vi "DCA Calibration Dialog.vi"(6 "Driver Refs":T4, 8 "error in (no error)":errorcluster, 11 "Current Calibration":T1) -> (0 "error out":errorcluster, 3 "Calibration Out":T1, 4 "Driver Refs Out":T4)   [LabVIEW 2011]
uses:
  drivers/DMM/DMM Driver Ref.ctl
  drivers/SWI/SWI Driver Ref.ctl
  TypeDefs/DCA Calibration State.ctl
  drivers/DMM/DMM Measurement.ctl
  drivers/DMM/DMM Command.ctl
  drivers/SWI/SWI Command.ctl
panel:
  out "Rbc Indicator":cluster{"Pass":bool, "Fail":bool}
  out "Rac Indicator":cluster{"Pass":bool, "Fail":bool}
  out "Rab Indicator":cluster{"Pass":bool, "Fail":bool}
  in  "Clear":bool
  in  "Rbc":bool
  in  "Rac":bool
  in  "Rab":bool
  in  "Done":bool
  in  "Message (\"\")":string="The instrument is ready for normalization.\n\nPlease insert the appropriate shorts into the test fixture and select one of the following options:\n\n    Rab  -  calibrate the Rab switch position.\n    Rac  -  calibrate the Rac switch position.\n    Rbc  -  calibrate the Rbc switch position.\n    Done  -  accept the normalization offsets and continue testing by\n                  following these steps:\n                     1)  Remove the short from the test fixtrue;\n                     2)  Place the part to be measured into the test fixture;\n                     3)  Press the Done button to continue."
  out "Cal Header":string="Normalization Offsets:\n\nRab = 0.00\nRac = 0.00\nRbc = 0.00"
  out "Cal Accepted?":bool
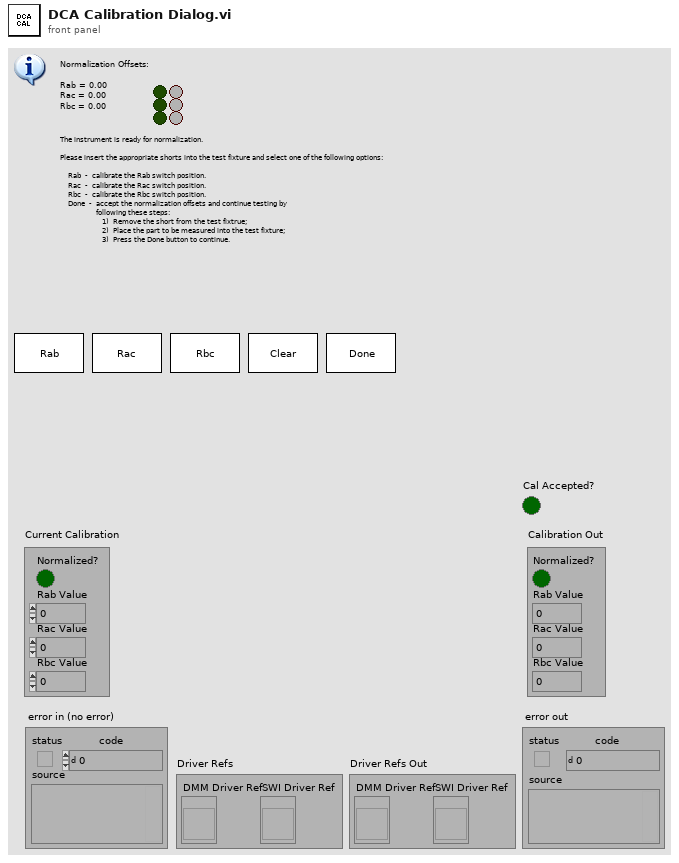
[diagram p1: front panel]
types:
  T1 = typedef "DCA Calibration State.ctl" = cluster{"Normalized?":bool, "Rab Value":dbl, "Rac Value":dbl, "Rbc Value":dbl}
  T2 = typedef "DMM Driver Ref.ctl" = refnum<vi>
  T3 = typedef "SWI Driver Ref.ctl" = refnum<vi>
  T4 = cluster{"DMM Driver Ref":T2, "SWI Driver Ref":T3}
  T5 = typedef "DMM Measurement.ctl" = dbl
  T6 = typedef "DMM Command.ctl" = enum16{"LOAD", "INITIALIZE", "PRESET", "GET STIMULUS", "SET STIMULUS", "MEASURE", "RELEASE", "UNLOAD", "GET CALIBRATION", "CALIBRATE"}
  T7 = typedef "SWI Command.ctl" = enum16{"LOAD", "INITIALIZE", "PRESET", "SET STIMULUS", "GET STIMULUS", "GET INFO", "RELEASE", "UNLOAD"}
  T8 = typedef "Sea-Level SWI Position.ctl" = cluster{"Port 1 (0)":cluster{"0":bool, "1":bool, "2":bool, "3":bool, "4":bool, "5":bool, "6":bool, "7":bool}, "Port 2 (1)":cluster{"0":bool, "1":bool, "2":bool, "3":bool, "4":bool, "5":bool, "6":bool, "7":bool}, "Port 3 (2)":cluster{"0":bool, "1":bool, "2":bool, "3":bool, "4":bool, "5":bool, "6":bool, "7":bool}, "Port 4 (3)":cluster{"0":bool, "1":bool, "2":bool, "3":bool, "4":bool, "5":bool, "6":bool, "7":bool}}
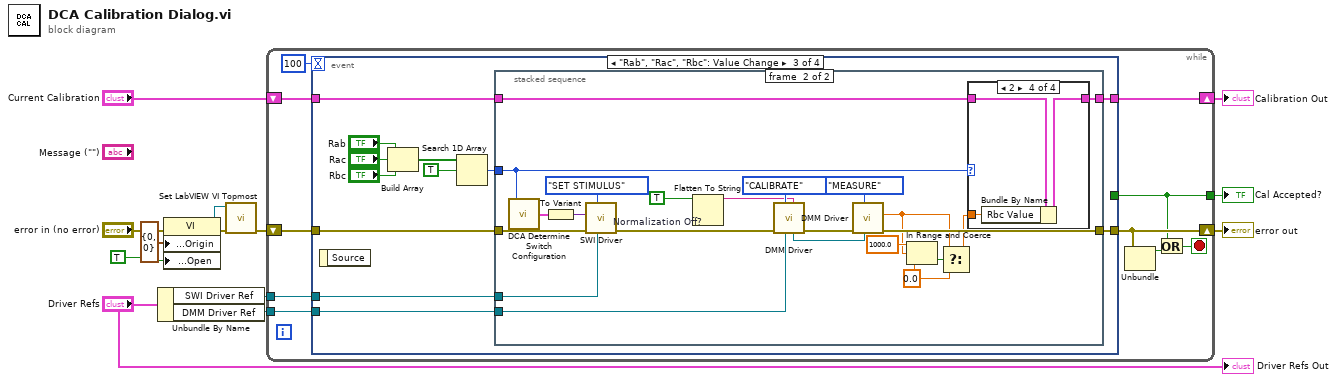
[diagram p0: block diagram]
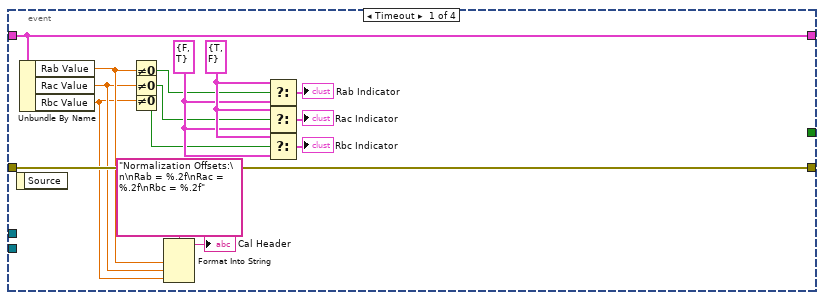
[diagram p2: hidden frame]
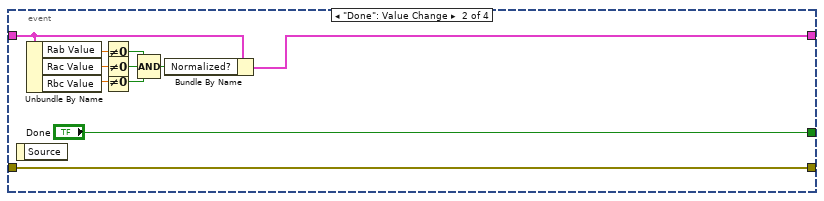
[diagram p3: hidden frame]
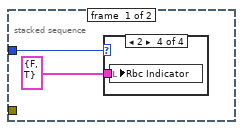
[diagram p4: hidden frame]
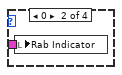
[diagram p6: hidden frame]
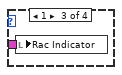
[diagram p7: hidden frame]
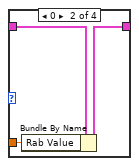
[diagram p9: hidden frame]
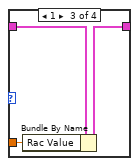
[diagram p10: hidden frame]
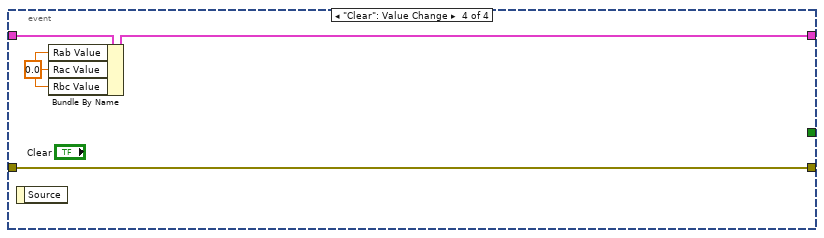
[diagram p11: hidden frame]
diagram:
  n1 = Unbundle By Name("Driver Refs") -> ("SWI Driver Ref"=w11:T3, "DMM Driver Ref"=w10:T2)
  n2 = property on="Property Node" class="VI"(error in="error in (no error)", "Front Panel Window:Origin"=cluster{"Horizontal":i16, "Vertical":i16} {"Horizontal"=0, "Vertical"=0}, "Front Panel Window:Open"=TRUE) -> (reference out=w6:refnum<vi>, error out=w5:errorcluster)  [unwired: 1 in]
  n3 = call "Set LabVIEW VI Topmost.vi"("error in (no error)"=w5, "VI Refnum (null)"=w6) -> ("error out"=w3:errorcluster)  [unwired: 7 in, 2 out]
  n4 = while {
    tunnel: [w14] -> w13
    tunnel: w11 -> [w23]
    tunnel: w10 -> [w22]
    shift-right: [w21] -> w1
    shift-left: "Current Calibration" -> [w20]
    shift-right: [w17] -> w12
    shift-left: w3 -> [w19]
    stop <- w16 stop-if-true
    n5 = event shown="[2] \"Rab\", \"Rac\", \"Rbc\": Value Change" {
      selector: _ -> [_ _ _ _]
      dyn-events: _ -> [_ _ _ _]
      timeout: 100 -> [_ _ _ _]
      tunnel: w19 -> [w36 w49 w61 w100]
      tunnel: [w36 w49 w56 w100] -> w17
      tunnel: w23 -> [_ _ w60 _]
      tunnel: w22 -> [_ _ w59 _]
      tunnel: w20 -> [w35 w45 w58 w102]
      tunnel: [w35 w47 w57 w101] -> w21
      tunnel: [_ "Done" _ _] -> w14
      event Timeout {
        w30 = cluster{"Pass":bool, "Fail":bool} {"Pass"=FALSE, "Fail"=TRUE} ("Rab Indicator")
        w31 = cluster{"Pass":bool, "Fail":bool} {"Pass"=TRUE, "Fail"=FALSE} ("Rab Indicator")
        n6 = event-data() -> ()  [unwired: 2 out]
        n7 = Unbundle By Name(w35) -> ("Rab Value"=w26:dbl, "Rac Value"=w25:dbl, "Rbc Value"=w24:dbl)
        n8 = Not Equal To 0?(x=w26) -> (x != 0?=w27:bool)
        n9 = Not Equal To 0?(x=w25) -> (x != 0?=w28:bool)
        n10 = Not Equal To 0?(x=w24) -> (x != 0?=w29:bool)
        n11 = Format Into String(format string="Normalization Offsets:\n\nRab = %.2f\nRac = %.2f\nRbc = %.2f", w26, w25, w24) -> (resulting string=→"Cal Header":string)  [unwired: 2 in, 1 out]
        n12 = Select(t=w31, s=w27, f=w30) -> (s? t:f=→"Rab Indicator":cluster{"Pass":bool, "Fail":bool})
        n13 = Select(t=w31, s=w28, f=w30) -> (s? t:f=→"Rac Indicator":cluster{"Pass":bool, "Fail":bool})
        n14 = Select(t=w31, s=w29, f=w30) -> (s? t:f=→"Rbc Indicator":cluster{"Pass":bool, "Fail":bool})
      }
      event "Done": Value Change {
        n15 = event-data() -> ()  [unwired: 2 out]
        n16 = Unbundle By Name(w45) -> ("Rab Value"=w41:dbl, "Rac Value"=w44:dbl, "Rbc Value"=w42:dbl)
        n17 = Not Equal To 0?(x=w41) -> (x != 0?=w40:bool)
        n18 = Not Equal To 0?(x=w44) -> (x != 0?=w43:bool)
        n19 = Not Equal To 0?(x=w42) -> (x != 0?=w39:bool)
        n20 = Compound Arithmetic op=AND(w40, w43, w39) -> (w46:bool)
        n21 = Bundle By Name(cluster=w45, "Normalized?"=w46) -> (w47:T1)
      }
      event "Rab", "Rac", "Rbc": Value Change {
        n22 = event-data() -> ()  [unwired: 2 out]
        n23 = Build Array("Rab", "Rac", "Rbc") -> (w51:bool[])
        n24 = Search 1D Array(1D array=w51, element=TRUE) -> (index of element=w50:i32)  [unwired: 1 out]
        n25 = stacked-sequence {
          tunnel: w61 -> [_ w86]
          tunnel: w60 -> [_ w85]
          tunnel: w59 -> [_ w81]
          tunnel: w58 -> [_ w79]
          tunnel: [_ w78] -> w57
          tunnel: [_ w77] -> w56
          tunnel: w50 -> [w63 w68]
          frame #0 {
            n26 = case shown="2" w63 {
              tunnel: cluster{"Pass":bool, "Fail":bool} {"Pass"=FALSE, "Fail"=TRUE} ("Rac Indicator") -> [_ w64 w65 w66]
              frame Default {
              }
              frame 0 {
                n27 = local write "Rab Indicator"(w64) -> ()
              }
              frame 1 {
                n28 = local write "Rac Indicator"(w65) -> ()
              }
              frame 2 {
                n29 = local write "Rbc Indicator"(w66) -> ()
              }
            }
          }
          frame #1 {
            w69 = T5 0.0 ("f")
            w76 = TRUE  # Normalization Off?
            n30 = call "DCA Determine Switch Configuration.vi"("Measurement"=w68) -> ("SWI Position"=w88:T8)
            n31 = To Variant(anything=w88) -> (Variant=w67:variant)
            n32 = call "SWI Driver.vi"("Drv Refnum"=w85, "SWI Command"=SWI_Command."SET STIMULUS", "error in (no error)"=w86, "SWI Position In"=w67) -> ("error out"=w74:errorcluster)  [unwired: 1 in, 6 out]
            n33 = Flatten To String(anything=w76) -> (data string=w75:string)  [unwired: 1 in, 4 out]
            n34 = call "DMM Driver.vi"("DMM Configuration (\"\")"=w75, "Drv Refnum"=w81, "DMM Command"=DMM_Command."CALIBRATE" ("VNA Command"), "error in (no error)"=w74) -> ("error out"=w84:errorcluster, "dup Drv Refnum"=w80:T2)  [unwired: 3 in, 3 out]
            n35 = call "DMM Driver.vi"("Drv Refnum"=w80, "DMM Command"=DMM_Command."MEASURE" ("VNA Command"), "error in (no error)"=w84) -> ("error out"=w77:errorcluster, "DMM Measurement"=w70:T5)  [unwired: 4 in, 3 out]
            n36 = In Range and Coerce(upper limit=T5 1000.0 ("y"), x=w70, lower limit=w69) -> (In Range?=w72:bool)  [unwired: 1 out]
            n37 = Select(t=w70, s=w72, f=w69) -> (s? t:f=w73:T5)
            n38 = case shown="2" w68 {
              tunnel: w79 -> [w89 w92 w95 w98]
              tunnel: [w89 w91 w94 w97] -> w78
              tunnel: w73 -> [_ w90 w93 w96]
              frame Default {
              }
              frame 0 {
                n39 = Bundle By Name(cluster=w92, "Rab Value"=w90) -> (w91:T1)
              }
              frame 1 {
                n40 = Bundle By Name(cluster=w95, "Rac Value"=w93) -> (w94:T1)
              }
              frame 2 {
                n41 = Bundle By Name(cluster=w98, "Rbc Value"=w96) -> (w97:T1)
              }
            }
          }
        }
      }
      event "Clear": Value Change {
        w99 = 0.0 ("Rac Value")
        n42 = event-data() -> ()  [unwired: 2 out]
        n43 = Bundle By Name(cluster=w102, "Rab Value"=w99, "Rac Value"=w99, "Rbc Value"=w99) -> (w101:T1)
      }
    }
    n44 = Unbundle(w17) -> ("status"=w15:bool)  [unwired: 2 out]
    n45 = Or(x=w14, y=w15) -> (x .or. y?=w16:bool)
  }
  "error out" <- w12
  "Cal Accepted?" <- w13
  "Calibration Out" <- w1
  "Driver Refs Out" <- "Driver Refs"
